vi "bronkhorst.vi"(0 "ALR_ON_OFF":T1, 1 "TMP_val":T3, 5 "ZY_control":T10 {"Y_H" step=1.0; "SP" step=0.01 format="%.2f"}, 7 "Z_ASetState":T11, 9 "Y_ASetState":T2=enum."auto", 11 "error in (no error)":errorcluster) -> (4 "ALR_ON_OFF out":T1, 6 "ZY_State":T12={"Z"={"Z_Source"=enum."initialize", "Z_SetState"=enum."initialization", "Z_State"=enum."initialization", "Z_State_T"=0, "ALR  L1"=FALSE, "ALR  L2"=FALSE, "HH_run"=0}, "Y"={"Y_Source"=enum."initialize", "Y_SetState"=enum."initialize", "SP_Set"=0.0, "SP"=0.0, "PV"=0.0, "PV_State"={"code"=0, "visible"=FALSE, "color"=0}, "Y_preSet"=0.0, "Y_Set"=0.0, "Y"=0.0, "Y_State"={"code"=0, "visible"=FALSE, "color"=0}, "YB"=FALSE}, "ALR_Status"=[], "control param"={"proportional gain (Kc)"=1.0, "integral time (Ti, s)"=10.0, "derivative time (Td, s)"=1.0, "output high"=100.0, "output high start"=40.0, "output high stop"=40.0, "alr value"=0.0, "output low"=0.0, "output rate (EGU/s)"=5.0, "setpoint max"=100.0, "setpoint rate (EGU/min)"=10.0, "stop rate (EGU/min)"=5.0}} {"control param"."setpoint max" format="%.2f"; "control param"."stop rate (EGU/min)" min=0.001 format="%.2f"; "control param"."setpoint rate (EGU/min)" min=0.001 format="%.2f"; "control param"."output high stop" format="%.2f"; "control param"."output high start" format="%.2f"; "control param"."output rate (EGU/s)" min=0.001 format="%.2f"; "control param"."output low" format="%.2f"; "control param"."alr value" format="%.2f"; "control param"."output high" format="%.2f"; "control param"."derivative time (Td, s)" format="%.3f"; "control param"."integral time (Ti, s)" format="%.3f"; "control param"."proportional gain (Kc)" format="%.3f"; "Y"."Y" format="%.2f"; "Y"."Y_preSet" format="%.2f"; "Y"."SP" step=0.01 format="%.2f"; "Y"."Y_Set" format="%.2f"; "Y"."PV" step=0.01 format="%.2f"; "Y"."SP_Set" step=0.01 format="%.2f"}, 8 "Y":dbl format="%.2f", 10 "ALR_L1":bool, 14 "YB":bool, 15 "error out":errorcluster)   [LabVIEW 2019]
uses:
  ctl/Z_State.ctl
  ctl/ZY_state_short.ctl
  ctl/Z.ctl
  Heating/ctl/Y_source.ctl
  Heating/ctl/Z_State.ctl
  ctl/Y_short.ctl
  ctl/Y_source.ctl
  ctl/Y_state.ctl
  Inputs/Ctl/Parameter State short.ctl
  Alarms/Ctl/ALR_Status_short.ctl
  ctl/control param.ctl
  Heating/ctl/ZY_control.ctl
  Heating/ctl/TMP_val.ctl
  Inputs/Ctl/Parameter State.ctl
  Alarms/Ctl/ALRs_State.ctl
  Alarms/Ctl/ALR_ON_OFF.ctl
  Alarms/Ctl/ALR_Parameters.ctl
  Alarms/Ctl/ALR code.ctl
  Alarms/Ctl/ALR type.ctl
  projects/Additivs/Regulators/PROG/GM1_201007/enums/System.ctl
  projects/Additivs/Regulators/PROG/GM1_201007/enums/PAR.ctl
  projects/Additivs/Regulators/PROG/GM1_201007/enums/AI.ctl
  projects/Additivs/Regulators/PROG/GM1_201007/enums/DI.ctl
  Heating/Z_switch_heating.vi
  Z_State_reg.vi
  Sequence/State1.vi
  Trigers/RS.vi
  Timer Delay/Timer.vi
  projects/Additivs/Regulators/PROG/GM1_201007/enums/Param_h0gm1.lvlib
  Heating/Heating.lvlib
  Alarms/Alarms.lvlib
  Inputs/Inputs.lvlib
  control.lvlib
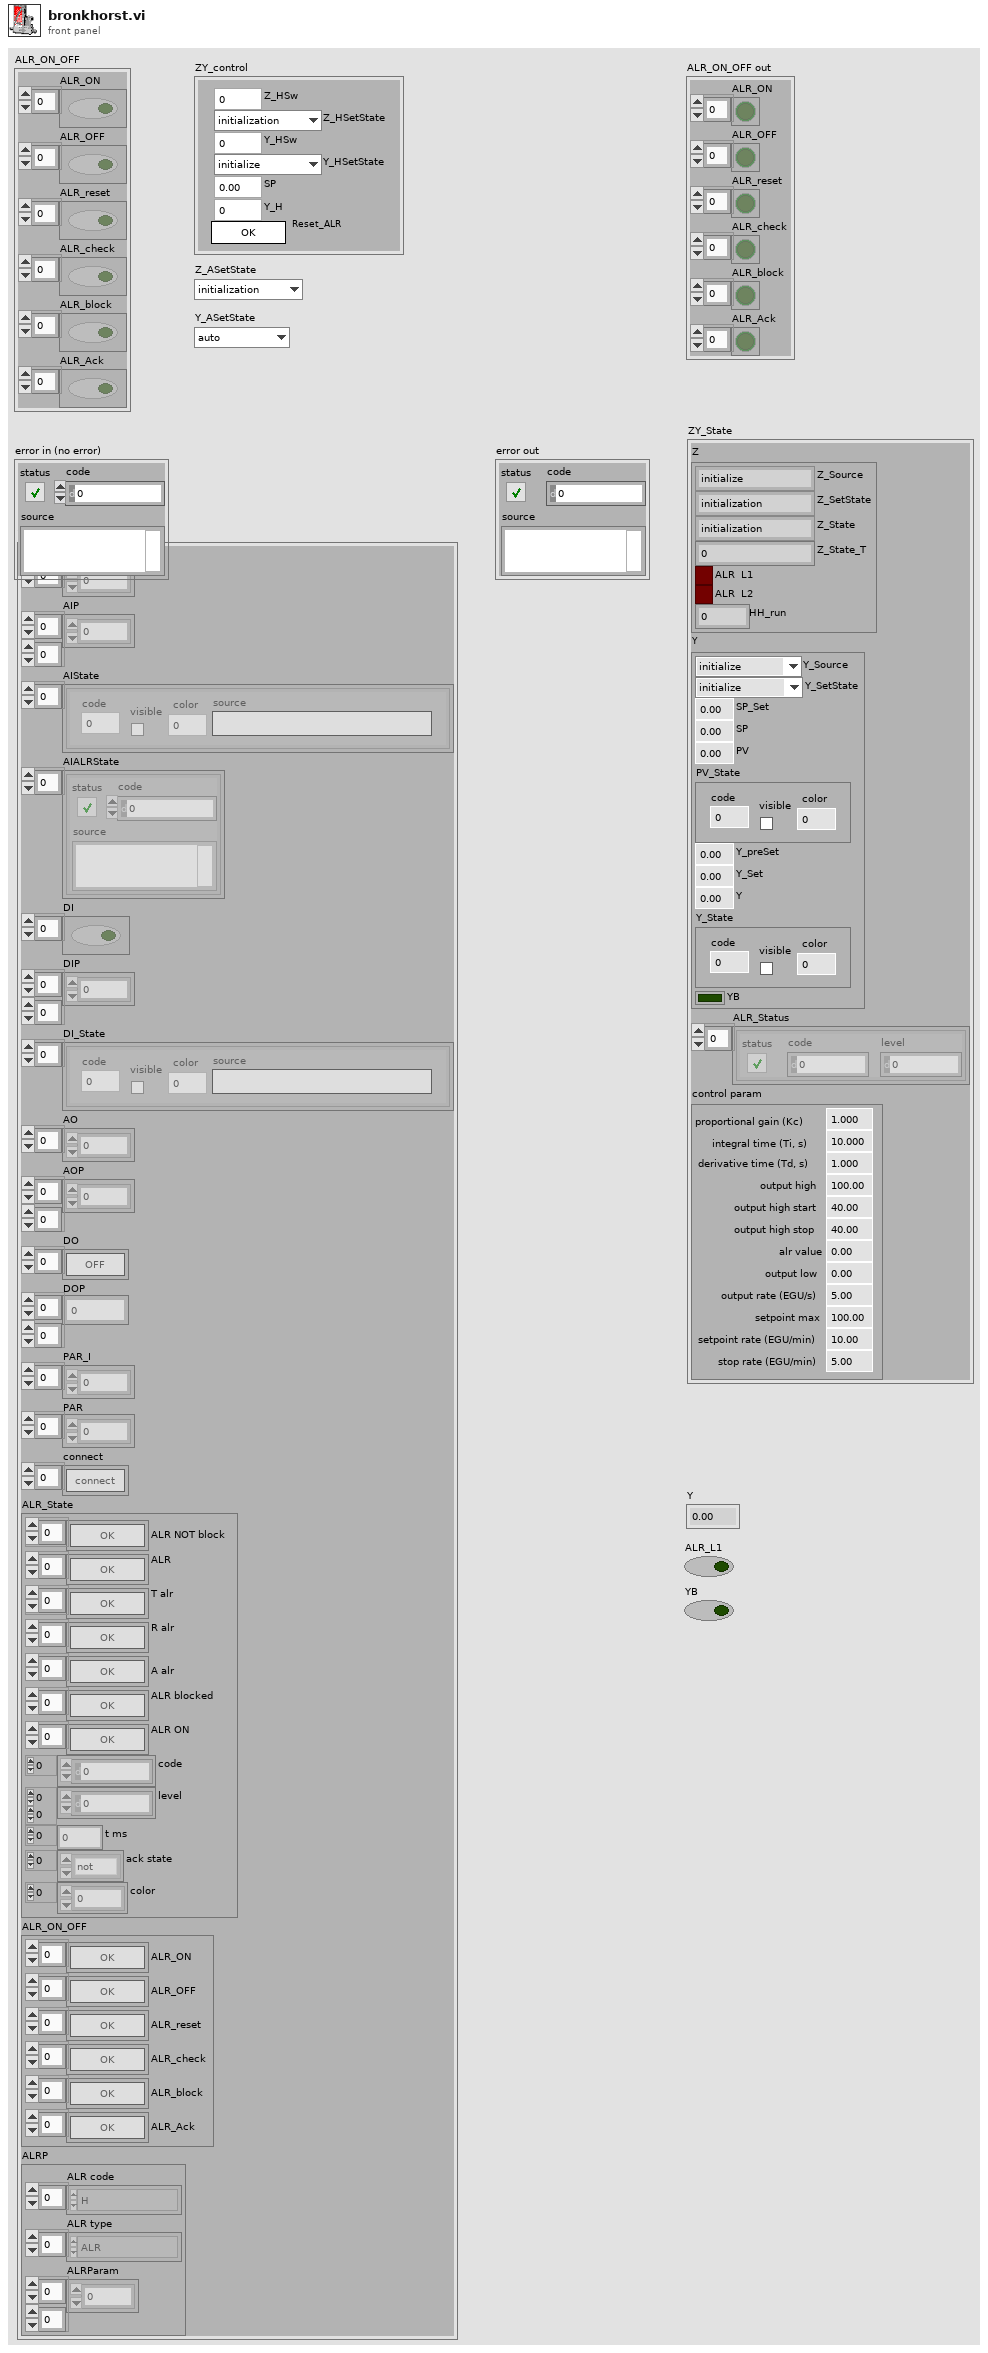
[diagram p1: front panel]
types:
  T1 = cluster{"ALR_ON":bool[], "ALR_OFF":bool[], "ALR_reset":bool[], "ALR_check":bool[], "ALR_block":bool[], "ALR_Ack":bool[]}
  T2 = typedef "control.lvlib/Y_state.ctl" = enum8{"initialize", "alarm", "min", "stop", "hand", "auto", "max"}
  T3 = typedef "Heating.lvlib/TMP_val.ctl" = cluster{"AI":dbl[], "AIP":dbl[][], "AIState":T4[], "AIALRState":errorcluster[], "DI":bool[], "DIP":dbl[][], "DI_State":T4[], "AO":dbl[], "AOP":dbl[][], "DO":bool[], "DOP":i32[][], "PAR_I":i32[], "PAR":dbl[], "connect":bool[], "ALR_State":T5, "ALR_ON_OFF":T6, "ALRP":T7}
  T4 = typedef "Inputs.lvlib/Parameter State.ctl" = cluster{"code":i32, "visible":bool, "color":u32, "source":string}
  T5 = typedef "Alarms.lvlib/ALRs_State.ctl" = cluster{"ALR NOT block":bool[], "ALR":bool[], "T alr":bool[], "R alr":bool[], "A alr":bool[], "ALR blocked":bool[], "ALR ON":bool[], "code":i32[], "level":i32[][], "t ms":u32[], "ack state":enum32{"not", "tripped", "reset", "ack"}[], "color":u32[]}
  T6 = typedef "Alarms.lvlib/ALR_ON_OFF.ctl" = cluster{"ALR_ON":bool[], "ALR_OFF":bool[], "ALR_reset":bool[], "ALR_check":bool[], "ALR_block":bool[], "ALR_Ack":bool[]}
  T7 = typedef "Alarms.lvlib/ALR_Parameters.ctl" = cluster{"ALR code":T8[], "ALR type":T9[], "ALRParam":u32[][]}
  T8 = typedef "Alarms.lvlib/ALR code.ctl" = enum16{"CONN", "H", "HH", "L", "LL", "SERR", "ON", "OFF", "XM19", "XM24", "XM47", "XM51", "XM52", "XM53", "XM54", "XM55", "XM56", "XM61", "XM62", "XM63", "XM64", "XM65", "XM66"}
  T9 = typedef "Alarms.lvlib/ALR type.ctl" = enum16{"ACD", "ACDR", "ALRN", "ALR"}
  T10 = typedef "Heating.lvlib/ZY_control.ctl" = cluster{"Z_HSw":u32, "Z_HSetState":T11, "Y_HSw":u32, "Y_HSetState":T2, "SP":dbl, "Y_H":dbl, "Reset_ALR":bool}
  T11 = typedef "control.lvlib/Z_State.ctl" = enum8{"initialization", "alarm", "disabled", "not ready", "stop ready", "reserv", "switched off", "reserv2", "switched on", "check", "on min", "decrease out", "on", "increase out", "on max"}
  T12 = typedef "ZY_state_short.ctl" = cluster{"Z":T13, "Y":T16, "ALR_Status":T19[], "control param":T20}
  T13 = typedef "Z.ctl" = cluster{"Z_Source":T14, "Z_SetState":T15, "Z_State":T15, "Z_State_T":u32, "ALR  L1":bool, "ALR  L2":bool, "HH_run":i32}
  T14 = typedef "Heating.lvlib/Y_source.ctl" = enum8{"initialize", "local disabled", "local hand", "hand", "auto", "dist"}
  T15 = typedef "Heating.lvlib/Z_State.ctl" = enum8{"initialization", "alarm", "disabled", "not ready", "stop ready", "reserv", "switched off", "reserv2", "switched on", "check", "on min", "decrease out", "on", "increase out", "on max"}
  T16 = typedef "control.lvlib/Y_short.ctl" = cluster{"Y_Source":T17, "Y_SetState":T2, "SP_Set":dbl, "SP":dbl, "PV":dbl, "PV_State":T18, "Y_preSet":dbl, "Y_Set":dbl, "Y":dbl, "Y_State":T18, "YB":bool}
  T17 = typedef "control.lvlib/Y_source.ctl" = enum8{"initialize", "local disabled", "local hand", "hand", "auto", "dist"}
  T18 = typedef "Inputs.lvlib/Parameter State short.ctl" = cluster{"code":i32, "visible":bool, "color":u32}
  T19 = typedef "Alarms.lvlib/ALR_Status_short.ctl" = cluster{"status":bool, "code":i32, "level":i32}
  T20 = typedef "control param.ctl" = cluster{"proportional gain (Kc)":dbl, "integral time (Ti, s)":dbl, "derivative time (Td, s)":dbl, "output high":dbl, "output high start":dbl, "output high stop":dbl, "alr value":dbl, "output low":dbl, "output rate (EGU/s)":dbl, "setpoint max":dbl, "setpoint rate (EGU/min)":dbl, "stop rate (EGU/min)":dbl}
  T21 = cluster{"proportional gain (Kc)":dbl, "integral time (Ti, s)":dbl, "derivative time (Td, s)":dbl, "output high":dbl, "output high start":dbl, "output high stop":dbl, "alr value":dbl, "output low":dbl, "output rate (EGU/s)":dbl, "setpoint max":dbl, "setpoint rate (EGU/min)":dbl, "stop rate (EGU/min)":dbl}
  T22 = typedef "Param_h0gm1.lvlib/System.ctl" = enum16{"GM3HT1", "GM3HT2", "EB2TB1", "EB2TB2", "EB2TB3", "EB3TB1", "EB3TB2", "EB3TB3"}
  T23 = typedef "Param_h0gm1.lvlib/PAR.ctl" = enum16{"GM3.HT1.TB1_t_stage_stop", "GM3.HT1.TB1_t_check", "GM3.HT1.TB1_t_start_delay", "GM3.HT1.TB1_t_heat_start", "GM3.HT1.TB1_t_stop_delay", "GM3.HT1.TB1_t_set_min", "GM3.HT1.TB1_t_heat_stop", "GM3.HT1.TB1_t_restart_delay", "GM3.HT1.TB1_t_HH_run", "GM3.HT1.TB1_pid_Kp", "GM3.HT1.TB1_pid_Ti", "GM3.HT1.TB1_pid_Td", "GM3.HT1.TB1_pid_output_high", "GM3.HT1.TB1_pid_out_start_H", "GM3.HT1.TB1_pid_out_stop_H", "GM3.HT1.TB1_pid_alr_value", "GM3.HT1.TB1_pid_output_low", "GM3.HT1.TB1_pid_setpoint_max", "GM3.HT1.TB1_pid_setpnt_rate", "GM3.HT1.TB1_pid_stop_rate", "GM3.HT1.TB1_pid_output_rate", "GM3.HT1.TB2_t_stage_stop", "GM3.HT1.TB2_t_check", "GM3.HT1.TB2_t_start_delay", "GM3.HT1.TB2_t_heat_start", "GM3.HT1.TB2_t_stop_delay", "GM3.HT1.TB2_t_set_min", "GM3.HT1.TB2_t_heat_stop", "GM3.HT1.TB2_t_restart_delay", "GM3.HT1.TB2_t_HH_run", "GM3.HT1.TB2_pid_Kp", "GM3.HT1.TB2_pid_Ti", "GM3.HT1.TB2_pid_Td", "GM3.HT1.TB2_pid_output_high", "GM3.HT1.TB2_pid_out_start_H", "GM3.HT1.TB2_pid_out_stop_H", "GM3.HT1.TB2_pid_alr_value", "GM3.HT1.TB2_pid_output_low", "GM3.HT1.TB2_pid_setpoint_max", "GM3.HT1.TB2_pid_setpnt_rate", "GM3.HT1.TB2_pid_stop_rate", "GM3.HT1.TB2_pid_output_rate", "GM3.1.BW1_u_ext", "GM3.1.BW1_t_weight", "GM3.1.MA1_t_stage_stop", "GM3.1.MA1_t_check", "GM3.1.MA1_t_start_delay", "GM3.1.MA1_t_start", "GM3.1.MA1_t_stop_delay", "GM3.1.MA1_t_set_min", "GM3.1.MA1_t_stop", "GM3.1.MA1_t_restart_delay", "GM3.1.MA1_t_max_on_right", "GM3.1.MA1_t_max_on_left", "GM3.1.MA1_t_HH_run", "GM3.1.MA1_pid_Kp", "GM3.1.MA1_pid_Ti", "GM3.1.MA1_pid_Td", "GM3.1.MA1_pid_output_high", "GM3.1.MA1_pid_out_start_H", "GM3.1.MA1_pid_out_stop_H", "GM3.1.MA1_pid_alr_value", "GM3.1.MA1_pid_output_low", "GM3.1.MA1_pid_output_rate", "GM3.1.MA1_pid_setpoint_max", "GM3.1.MA1_pid_setpnt_rate", "GM3.1.MA1_pid_stop_rate", "GM3.1.MA2_t_stage_stop", "GM3.1.MA2_t_check", "GM3.1.MA2_t_start_delay", "GM3.1.MA2_t_start", "GM3.1.MA2_t_stop_delay", "GM3.1.MA2_t_set_min", "GM3.1.MA2_t_stop", "GM3.1.MA2_t_restart_delay", "GM3.1.MA2_t_max_on_right", "GM3.1.MA2_t_max_on_left", "GM3.1.MA2_pid_output_high", "GM3.1.QM5_t_on", "GM3.1.QM5_t_off", "GM3.2.MA1_t_stage_stop", "GM3.2.MA1_t_check", "GM3.2.MA1_t_start_delay", "GM3.2.MA1_t_start", "GM3.2.MA1_t_stop_delay", "GM3.2.MA1_t_set_min", "GM3.2.MA1_t_stop", "GM3.2.MA1_t_restart_delay", "GM3.2.MA1_t_max_on_right", "GM3.2.MA1_t_max_on_left", "GM3.2.MA1_pid_output_high", "GM3.2.MA2_t_stage_stop", "GM3.2.MA2_t_check", "GM3.2.MA2_t_start_delay", "GM3.2.MA2_t_start", "GM3.2.MA2_t_stop_delay", "GM3.2.MA2_t_set_min", "GM3.2.MA2_t_stop", "GM3.2.MA2_t_restart_delay", "GM3.2.MA2_t_max_on_right", "GM3.2.MA2_t_max_on_left", "GM3.2.MA2_pid_output_high", "EB2.TB.1_t_stage_stop", "EB2.TB.1_t_check", "EB2.TB.1_t_start_delay", "EB2.TB.1_t_heat_start", "EB2.TB.1_t_stop_delay", "EB2.TB.1_t_set_min", "EB2.TB.1_t_heat_stop", "EB2.TB.1_t_restart_delay", "EB2.TB.1_t_HH_run", "EB2.TB.1_pid_Kp", "EB2.TB.1_pid_Ti", "EB2.TB.1_pid_Td", "EB2.TB.1_pid_output_high", "EB2.TB.1_pid_out_start_H", "EB2.TB.1_pid_out_stop_H", "EB2.TB.1_pid_alr_value", "EB2.TB.1_pid_output_low", "EB2.TB.1_pid_setpoint_max", "EB2.TB.1_pid_setpnt_rate", "EB2.TB.1_pid_stop_rate", "EB2.TB.1_pid_output_rate", "EB2.TB.2_t_stage_stop", "EB2.TB.2_t_check", "EB2.TB.2_t_start_delay", "EB2.TB.2_t_heat_start", "EB2.TB.2_t_stop_delay", "EB2.TB.2_t_set_min", "EB2.TB.2_t_heat_stop", "EB2.TB.2_t_restart_delay", "EB2.TB.2_t_HH_run", "EB2.TB.2_pid_Kp", "EB2.TB.2_pid_Ti", "EB2.TB.2_pid_Td", "EB2.TB.2_pid_output_high", "EB2.TB.2_pid_out_start_H", "EB2.TB.2_pid_out_stop_H", "EB2.TB.2_pid_alr_value", "EB2.TB.2_pid_output_low", "EB2.TB.2_pid_setpoint_max", "EB2.TB.2_pid_setpnt_rate", "EB2.TB.2_pid_stop_rate", "EB2.TB.2_pid_output_rate", "EB2.TB.3_t_stage_stop", "EB2.TB.3_t_check", "EB2.TB.3_t_start_delay", "EB2.TB.3_t_heat_start", "EB2.TB.3_t_stop_delay", "EB2.TB.3_t_set_min", "EB2.TB.3_t_heat_stop", "EB2.TB.3_t_restart_delay", "EB2.TB.3_t_HH_run", "EB2.TB.3_pid_Kp", "EB2.TB.3_pid_Ti", "EB2.TB.3_pid_Td", "EB2.TB.3_pid_output_high", "EB2.TB.3_pid_out_start_H", "EB2.TB.3_pid_out_stop_H", "EB2.TB.3_pid_alr_value", "EB2.TB.3_pid_output_low", "EB2.TB.3_pid_setpoint_max", "EB2.TB.3_pid_setpnt_rate", "EB2.TB.3_pid_stop_rate", "EB2.TB.3_pid_output_rate", "EB3.TB.1_t_stage_stop", "EB3.TB.1_t_check", "EB3.TB.1_t_start_delay", "EB3.TB.1_t_heat_start", "EB3.TB.1_t_stop_delay", "EB3.TB.1_t_set_min", "EB3.TB.1_t_heat_stop", "EB3.TB.1_t_restart_delay", "EB3.TB.1_t_HH_run", "EB3.TB.1_pid_Kp", "EB3.TB.1_pid_Ti", "EB3.TB.1_pid_Td", "EB3.TB.1_pid_output_high", "EB3.TB.1_pid_out_start_H", "EB3.TB.1_pid_out_stop_H", "EB3.TB.1_pid_alr_value", "EB3.TB.1_pid_output_low", "EB3.TB.1_pid_setpoint_max", "EB3.TB.1_pid_setpnt_rate", "EB3.TB.1_pid_stop_rate", "EB3.TB.1_pid_output_rate", "EB3.TB.2_t_stage_stop", "EB3.TB.2_t_check", "EB3.TB.2_t_start_delay", "EB3.TB.2_t_heat_start", "EB3.TB.2_t_stop_delay", "EB3.TB.2_t_set_min", "EB3.TB.2_t_heat_stop", "EB3.TB.2_t_restart_delay", "EB3.TB.2_t_HH_run", "EB3.TB.2_pid_Kp", "EB3.TB.2_pid_Ti", "EB3.TB.2_pid_Td", "EB3.TB.2_pid_output_high", "EB3.TB.2_pid_out_start_H", "EB3.TB.2_pid_out_stop_H", "EB3.TB.2_pid_alr_value", "EB3.TB.2_pid_output_low", "EB3.TB.2_pid_setpoint_max", "EB3.TB.2_pid_setpnt_rate", "EB3.TB.2_pid_stop_rate", "EB3.TB.2_pid_output_rate", "EB3.TB.3_t_stage_stop", "EB3.TB.3_t_check", "EB3.TB.3_t_start_delay", "EB3.TB.3_t_heat_start", "EB3.TB.3_t_stop_delay", "EB3.TB.3_t_set_min", "EB3.TB.3_t_heat_stop", "EB3.TB.3_t_restart_delay", "EB3.TB.3_t_HH_run", "EB3.TB.3_pid_Kp", "EB3.TB.3_pid_Ti", "EB3.TB.3_pid_Td", "EB3.TB.3_pid_output_high", "EB3.TB.3_pid_out_start_H", "EB3.TB.3_pid_out_stop_H", "EB3.TB.3_pid_alr_value", "EB3.TB.3_pid_output_low", "EB3.TB.3_pid_setpoint_max", "EB3.TB.3_pid_setpnt_rate", "EB3.TB.3_pid_stop_rate", "EB3.TB.3_pid_output_rate"}
  T24 = typedef "Param_h0gm1.lvlib/AI.ctl" = enum16{"EB2.BC11", "EB2.BC12", "EB2.BC21", "EB2.BC22", "EB2.BP1", "EB2.BT1", "EB2.BT2", "EB2.BT3", "EB2.BT4", "EB2.BT5", "EB2.QN1", "EB2.QN2", "EB2.TB.1_BA1", "EB2.TB.1_BC1", "EB2.TB.1_BE1", "EB2.TB.1_BJ1", "EB2.TB.2_BA2", "EB2.TB.2_BC2", "EB2.TB.2_BE2", "EB2.TB.2_BJ2", "EB2.TB.3_BA3", "EB2.TB.3_BC3", "EB2.TB.3_BE3", "EB2.TB.3_BJ3", "EB2.TB_BJ", "EB2_BC1", "EB2_BC2", "EB3.BP1", "EB3.BT11", "EB3.BT12", "EB3.BT21", "EB3.BT22", "EB3.BT31", "EB3.BT32", "EB3.QN1", "EB3.QN2", "EB3.TB.1_BA1", "EB3.TB.1_BC1", "EB3.TB.1_BE1", "EB3.TB.1_BJ1", "EB3.TB.2_BA2", "EB3.TB.2_BC2", "EB3.TB.2_BE2", "EB3.TB.2_BJ2", "EB3.TB.3_BA3", "EB3.TB.3_BC3", "EB3.TB.3_BE3", "EB3.TB.3_BJ3", "EB3.TB_BJ", "EB3_BC1", "EB3_BC2", "GM2.EP1.BT1", "GM2.EP1.BT10", "GM2.EP1.BT11", "GM2.EP1.BT2", "GM2.EP1.BT3", "GM2.EP1.BT4", "GM2.EP1.BT5", "GM2.EP1.BT6", "GM2.EP1.BT7", "GM2.EP1.BT8", "GM2.EP1.BT9", "GM3.1.BP1", "GM3.1.BP2", "GM3.1.BW1", "GM3.1.BW1_BQ01", "GM3.1.BW1_BQ03", "GM3.1.BW1_XZ01", "GM3.1.BW2", "GM3.1.BW2_BQ01", "GM3.1.BW2_XZ01", "GM3.1.QN1", "GM3.2.BP1", "GM3.2.QN1", "GM3.2.QN2", "GM3.HT1.BC1", "GM3.HT1.BC2", "GM3.HT1.BT1", "GM3.HT1.BT2", "HW3.BT1", "HW3.BT2", "HW3.BT3"}
  T25 = typedef "Param_h0gm1.lvlib/DI.ctl" = enum16{"EB2.QM2_XB01", "EB2.QM2_XB24", "EB2.QM4_XB01", "EB2.QM4_XB24", "EB2.TB.1_XB01", "EB2.TB.1_XB02", "EB2.TB.1_XB19", "EB2.TB.1_XB47", "EB2.TB.2_XB01", "EB2.TB.2_XB02", "EB2.TB.2_XB19", "EB2.TB.2_XB47", "EB2.TB.3_XB01", "EB2.TB.3_XB02", "EB2.TB.3_XB19", "EB2.TB.3_XB47", "EB3.QM1_XB01", "EB3.QM1_XB24", "EB3.QM2_XB01", "EB3.QM2_XB24", "EB3.TB.1_XB01", "EB3.TB.1_XB02", "EB3.TB.1_XB19", "EB3.TB.1_XB47", "EB3.TB.2_XB01", "EB3.TB.2_XB02", "EB3.TB.2_XB19", "EB3.TB.2_XB47", "EB3.TB.3_XB01", "EB3.TB.3_XB02", "EB3.TB.3_XB19", "EB3.TB.3_XB47", "GM2.FZ1_XB19", "GM2.FZ2_XB21", "GM3.1.QM1_XB01", "GM3.1.QM1_XB24", "GM3.1.QM2_XB01", "GM3.1.QM2_XB24", "GM3.1.QM6_XB09", "GM3.1.QM6_XB10", "GM3.2.BG11_XB01", "GM3.2.BG12_XB01", "GM3.2.BG21_XB01", "GM3.2.BG22_XB01", "GM3.2.QM1_XB01", "GM3.2.QM1_XB24", "GM3.2.QM2_XB01", "GM3.2.QM2_XB24", "GM3.FZ1_XB19", "GM3.FZ2_XB21", "GM3.HT1.TB1_XB01", "GM3.HT1.TB2_XB01", "GM3.HT1_XB47"}
  T26 = cluster{"Z_HSw":u32, "Z_HSetState":T11, "Z_ASetState":T11, "Z_ASetState":T11}
  T27 = cluster{"Y_HSw":u32, "Y_HSetState":T2, "Y_ASetState":T2, "Y_ASetState":T2}
  T28 = typedef "Param_h0gm1.lvlib/ALR.ctl" = enum16{"EB2.BP1_H", "EB2.BP1_HH", "EB2.BP1_L", "EB2.BP1_SERR", "EB2.TB.1.2TB1_CONN", "EB2.TB.1.BA1_H", "EB2.TB.1.BC1_H", "EB2.TB.1.BC1_HH", "EB2.TB.1.BC1_L", "EB2.TB.1.BE1_H", "EB2.TB.1.BE1_HH", "EB2.TB.1.BE1_L", "EB2.TB.1.BE1_LL", "EB2.TB.2.2TB2_CONN", "EB2.TB.2.BA2_H", "EB2.TB.2.BC2_H", "EB2.TB.2.BC2_HH", "EB2.TB.2.BC2_L", "EB2.TB.2.BE2_H", "EB2.TB.2.BE2_HH", "EB2.TB.2.BE2_L", "EB2.TB.2.BE2_LL", "EB2.TB.3.2TB3_CONN", "EB2.TB.3.BA3_H", "EB2.TB.3.BC3_H", "EB2.TB.3.BC3_HH", "EB2.TB.3.BC3_L", "EB2.TB.3.BE3_H", "EB2.TB.3.BE3_HH", "EB2.TB.3.BE3_L", "EB2.TB.3.BE3_LL", "EB2.TF1.A13.1_CONN", "EB2.TF1.A13_CONN", "EB3.BP1_H", "EB3.BP1_HH", "EB3.BP1_L", "EB3.BP1_SERR", "EB3.BT11_H", "EB3.BT11_HH", "EB3.BT11_L", "EB3.BT11_SERR", "EB3.BT12_H", "EB3.BT12_HH", "EB3.BT12_L", "EB3.BT12_SERR", "EB3.BT21_H", "EB3.BT21_HH", "EB3.BT21_L", "EB3.BT21_SERR", "EB3.BT22_H", "EB3.BT22_HH", "EB3.BT22_L", "EB3.BT22_SERR", "EB3.BT31_H", "EB3.BT31_HH", "EB3.BT31_L", "EB3.BT31_SERR", "EB3.BT32_H", "EB3.BT32_HH", "EB3.BT32_L", "EB3.BT32_SERR", "EB3.TB.1.3TB1_CONN", "EB3.TB.1.BA1_H", "EB3.TB.1.BC1_H", "EB3.TB.1.BC1_HH", "EB3.TB.1.BC1_L", "EB3.TB.1.BE1_H", "EB3.TB.1.BE1_HH", "EB3.TB.1.BE1_L", "EB3.TB.1.BE1_LL", "EB3.TB.1_XM19", "EB3.TB.1_XM47", "EB3.TB.1_XM51", "EB3.TB.1_XM52", "EB3.TB.1_XM61", "EB3.TB.1_XM62", "EB3.TB.2.3TB2_CONN", "EB3.TB.2.BA2_H", "EB3.TB.2.BC2_H", "EB3.TB.2.BC2_HH", "EB3.TB.2.BC2_L", "EB3.TB.2.BE2_H", "EB3.TB.2.BE2_HH", "EB3.TB.2.BE2_L", "EB3.TB.2.BE2_LL", "EB3.TB.2_XM19", "EB3.TB.2_XM47", "EB3.TB.2_XM51", "EB3.TB.2_XM52", "EB3.TB.2_XM61", "EB3.TB.2_XM62", "EB3.TB.3.3TB3_CONN", "EB3.TB.3.BA3_H", "EB3.TB.3.BC3_H", "EB3.TB.3.BC3_HH", "EB3.TB.3.BC3_L", "EB3.TB.3.BE3_H", "EB3.TB.3.BE3_HH", "EB3.TB.3.BE3_L", "EB3.TB.3.BE3_LL", "EB3.TB.3_XM19", "EB3.TB.3_XM47", "EB3.TB.3_XM51", "EB3.TB.3_XM52", "EB3.TB.3_XM61", "EB3.TB.3_XM62", "GM2.EP1.BT1_H", "GM2.EP1.BT1_HH", "GM2.EP1.BT1_SERR", "GM2.EP1.BT10_H", "GM2.EP1.BT10_HH", "GM2.EP1.BT10_SERR", "GM2.EP1.BT11_H", "GM2.EP1.BT11_HH", "GM2.EP1.BT11_SERR", "GM2.EP1.BT2_H", "GM2.EP1.BT2_HH", "GM2.EP1.BT2_SERR", "GM2.EP1.BT3_H", "GM2.EP1.BT3_HH", "GM2.EP1.BT3_SERR", "GM2.EP1.BT4_H", "GM2.EP1.BT4_HH", "GM2.EP1.BT4_SERR", "GM2.EP1.BT5_H", "GM2.EP1.BT5_HH", "GM2.EP1.BT5_SERR", "GM2.EP1.BT6_H", "GM2.EP1.BT6_HH", "GM2.EP1.BT6_SERR", "GM2.EP1.BT7_H", "GM2.EP1.BT7_HH", "GM2.EP1.BT7_SERR", "GM2.EP1.BT8_H", "GM2.EP1.BT8_HH", "GM2.EP1.BT8_SERR", "GM2.EP1.BT9_H", "GM2.EP1.BT9_HH", "GM2.EP1.BT9_SERR", "GM2.FZ1_OFF", "GM2.FZ2_OFF", "GM2.KF1.A11_CONN", "GM2.KF1.A12_CONN", "GM2.KF1.A14_CONN", "GM2.KF1.A15_CONN", "GM2.KF1.A19_CONN", "GM2.TF3.A117_CONN", "GM2.TF3.A118_CONN", "GM3.1.BP1_H", "GM3.1.BP1_HH", "GM3.1.BP1_L", "GM3.1.BP1_SERR", "GM3.1.BP2_H", "GM3.1.BP2_HH", "GM3.1.BP2_L", "GM3.1.BP2_SERR", "GM3.1.QN1_L", "GM3.1.QN1_SERR", "GM3.2.QN2_L", "GM3.2.QN2_SERR", "GM3.FZ1_OFF", "GM3.FZ2_OFF", "GM3.HT1.BC1_SERR", "GM3.HT1.BC2_SERR", "GM3.HT1.BT1_H", "GM3.HT1.BT1_HH", "GM3.HT1.BT1_L", "GM3.HT1.BT1_SERR", "GM3.HT1.BT2_H", "GM3.HT1.BT2_HH", "GM3.HT1.BT2_L", "GM3.HT1.BT2_SERR", "GM3.HT1_XM47", "GM3.JBA1.A13_CONN", "GM3.KF1.A11_CONN", "GM3.KF1.A12_CONN", "GM3.KF1.A15_CONN", "GM3.KF1.A16_CONN", "GM3.KF1.A17_CONN", "GM3.KF1.A18_CONN", "GM3.KF1.A19_CONN", "GM3.TF1.A111_CONN", "GM3.TF1.A112_CONN", "GM3.TF1.A113_CONN", "GM3.TF1.A114_CONN", "GM3.TF1.A116_CONN", "GM3.TF1.A117_CONN", "GM3.TF1.A118_CONN", "GM3.TF1.A14_CONN", "HW2.TF1.A16_CONN", "HW3.BT1_H", "HW3.BT1_HH", "HW3.BT1_L", "HW3.BT1_SERR", "HW3.BT2_H", "HW3.BT2_HH", "HW3.BT2_L", "HW3.BT2_SERR", "HW3.BT3_H", "HW3.BT3_HH", "HW3.BT3_L", "HW3.BT3_SERR", "HX.TF1.A11_CONN", "HX.TF1.A14_CONN", "HX.TF2.A15_CONN"}
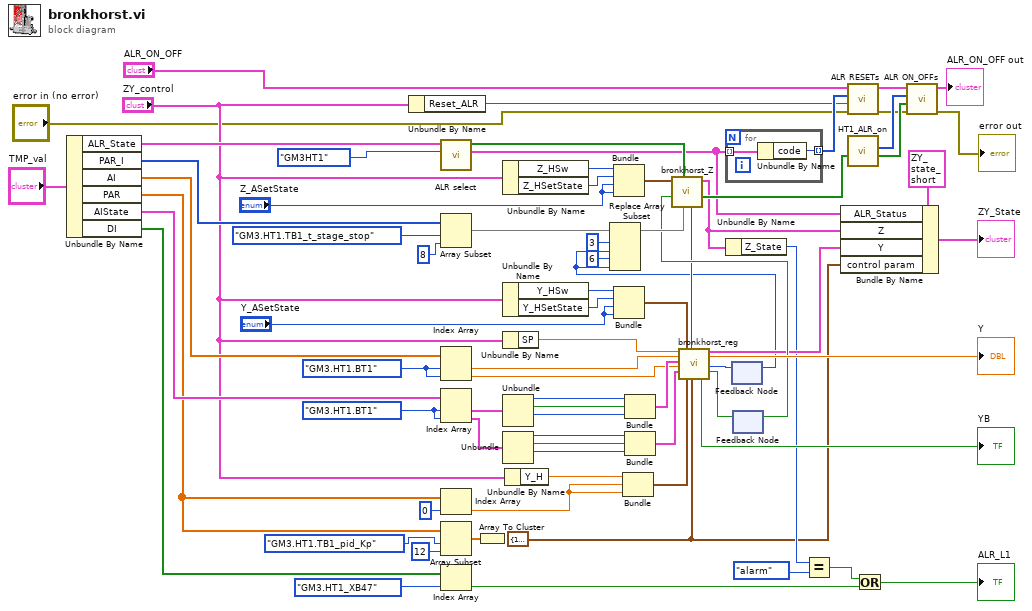
[diagram p0: block diagram]
diagram:
  w30 = T21 {"proportional gain (Kc)"=1.0, "integral time (Ti, s)"=10.0, "derivative time (Td, s)"=1.0, "output high"=100.0, "output high start"=40.0, "output high stop"=40.0, "alr value"=3.01, "output low"=0.0, "output rate (EGU/s)"=5.0, "setpoint max"=100.0, "setpoint rate (EGU/min)"=10.0, "stop rate (EGU/min)"=5.0} ("REG param")
  w19 = AI."GM3.HT1.BT1" ("AI 2")
  w21 = AI."GM3.HT1.BT1" ("AI 2")
  n1 = Unbundle By Name("TMP_val") -> ("ALR_State"=w48:T5, "PAR_I"=w47:i32[], "AI"=w46:dbl[], "PAR"=w25:dbl[], "AIState"=w45:T4[], "DI"=w44:bool[])
  n2 = Unbundle By Name("ZY_control") -> ("Reset_ALR"=w27:bool)
  n3 = call "ALR select.vi"("System"=System."GM3HT1" ("System_enum"), "ALR_State"=w48) -> ("ALR_Status"=w4:T19[], "ALRs"=w54:bool[])  [unwired: 8 in]
  n4 = Array Subset(array=w47, index=PAR."GM3.HT1.TB1_t_stage_stop" ("PAR"), length=8) -> (w58:i32[])
  n5 = Index Array(array=w46, index #1=w21, index #2=w21) -> (element #1=w75:dbl, element #2=w20:dbl)
  n6 = Index Array(array=w45, index #1=w19, index #2=w19) -> (element #1=w43:T4, element #2=w11:T4)
  n7 = Index Array(array=w25, index=0) -> (element=w22:dbl)
  n8 = Array Subset(array=w25, index=PAR."GM3.HT1.TB1_pid_Kp" ("PAR"), length=12) -> (w64:dbl[])
  n9 = Index Array(array=w44, index=DI."GM3.HT1_XB47" ("DI 2")) -> (element=w50:bool)
  n10 = Array To Cluster(array=w64) -> ()  [unwired: 1 out]
  n11 = Unbundle By Name("ZY_control") -> ("Z_HSw"=w9:u32, "Z_HSetState"=w8:T11)
  n12 = Unbundle By Name("ZY_control") -> ("Y_HSw"=w18:u32, "Y_HSetState"=w17:T2)
  n13 = Unbundle By Name("ZY_control") -> ("SP"=w28:dbl)
  n14 = Unbundle(w43) -> ("code"=w42:i32, "visible"=w41:bool, "color"=w40:u32)  [unwired: 1 out]
  n15 = Unbundle(w11) -> ("code"=w12:i32, "visible"=w13:bool, "color"=w14:u32)  [unwired: 1 out]
  n16 = Unbundle By Name("ZY_control") -> ("Y_H"=w29:dbl)
  n17 = Bundle("Z_HSw"=w9, "Z_HSetState"=w8, "Z_ASetState"="Z_ASetState", "Z_ASetState"="Z_ASetState") -> (w6:T26)  [unwired: 1 in]
  n18 = Bundle("Y_HSw"=w18, "Y_HSetState"=w17, "Y_ASetState"="Y_ASetState", "Y_ASetState"="Y_ASetState") -> (w15:T27)  [unwired: 1 in]
  n19 = Bundle("Y_H"=w29, "PAR"=w22, "PAR"=w22) -> (w23:cluster{"Y_H":dbl, "PAR":dbl, "PAR":dbl})  [unwired: 1 in]
  n20 = Bundle("code"=w42, "visible"=w41, "color"=w40) -> (w39:cluster{"code":i32, "visible":bool, "color":u32})  [unwired: 1 in]
  n21 = Bundle("code"=w12, "visible"=w13, "color"=w14) -> (w10:cluster{"code":i32, "visible":bool, "color":u32})  [unwired: 1 in]
  n22 = for {
    tunnel: w4 -> [w78] mode=indexing
    tunnel: [w77] -> w55 mode=indexing
    n23 = Unbundle By Name(w78) -> ("code"=w77:i32)
  }
  n24 = feedback #1() -> (w5:u32)  [unwired: 1 in]
  n25 = Replace Array Subset(array=w58, new element #1=w5, index #1=3 ("index"), new element #2=w5, index #2=6 ("index")) -> (w57:i32[])
  n26 = feedback #2() -> (w34:bool)  [unwired: 1 in]
  n27 = call "bronkhorst_Z.vi"("T"=w57, "Alarm"=w54, "ZB"=w34, "Z_in"=w6) -> ("ALR_ON"=w63:bool[], "Z"=w61:T13, "Z_State_next"=w31:u32)  [unwired: 5 in]
  n28 = call "bronkhorst_reg.vi"("SP"=w28, "PV"=w75, "PV_State"=w39, "Y"=w20, "Y_State"=w10, "Y_Set"=w15, "controls Y"=w23, "Z"=w31, "control param"=w30) -> ("YB"=→"YB":bool, "Y_State"=w33:T16, "Y"=→"Y":dbl, "T"=w74:u32, "End"=w35:bool)  [unwired: 6 in]
  n29 = Unbundle By Name(w61) -> ("Z_State"=w32:T15)
  n30 = feedback-in #1(w74) -> ()
  n31 = feedback-in #2(w35) -> ()
  n32 = Equal?(x=w32, y=Z_State."alarm" ("Z_State")) -> (x = y?=w52:bool)
  n33 = Bundle By Name(cluster=T12 {"Z"={"Z_Source"=enum."local disabled", "Z_SetState"=enum."on", "Z_State"=enum."alarm", "Z_State_T"=0, "ALR  L1"=FALSE, "ALR  L2"=FALSE, "HH_run"=0}, "Y"={"Y_Source"=enum."local disabled", "Y_SetState"=enum."auto", "SP_Set"=0.0, "SP"=0.0, "PV"=0.0, "PV_State"={"code"=0, "visible"=FALSE, "color"=0}, "Y_preSet"=0.0, "Y_Set"=0.0, "Y"=0.0, "Y_State"={"code"=0, "visible"=FALSE, "color"=0}, "YB"=FALSE}, "ALR_Status"=[], "control param"={"proportional gain (Kc)"=1.0, "integral time (Ti, s)"=10.0, "derivative time (Td, s)"=1.0, "output high"=100.0, "output high start"=40.0, "output high stop"=40.0, "alr value"=0.0, "output low"=0.0, "output rate (EGU/s)"=5.0, "setpoint max"=100.0, "setpoint rate (EGU/min)"=10.0, "stop rate (EGU/min)"=5.0}} ("ZY_State"), "ALR_Status"=w4, "Z"=w61, "Y"=w33, "control param"=w30) -> (→"ZY_State":T12)
  n34 = call "ALR RESETs.vi"("error in (no error)"="error in (no error)", "Reset"=w27, "Index"=w55, "ALR_ON_OFF"="ALR_ON_OFF") -> ("error out"=w37:errorcluster, "ALR_ON_OFF out"=w36:T6)  [unwired: 6 in]
  n35 = call "HT1_ALR_on.vi"("Data in"=w63) -> ("Data"=w62:bool[], "Index"=w59:T28[])  [unwired: 9 in]
  n36 = Or(x=w52, y=w50) -> (x .or. y?=→"ALR_L1":bool)
  n37 = call "ALR ON_OFFs.vi"("error in (no error)"=w37, "Data"=w62, "Index"=w59, "ALR_ON_OFF"=w36) -> ("error out"=→"error out":errorcluster, "ALR_ON_OFF out"=→"ALR_ON_OFF out":T6)  [unwired: 6 in]
